vi "make step function for duty cycle.vi"(7 "delay":dbl, 8 "amplitude":dbl, 9 "period":dbl, 10 "duty cycle":dbl, 11 "sample rate":dbl) -> (3 "Waveform out":waveform(dbl))   [LabVIEW 2025]
uses:
  <vilib>/Analysis/NI_AALBase.lvlib
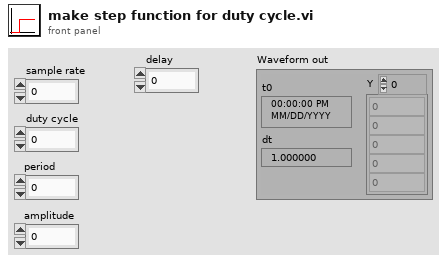
[diagram p1: front panel]
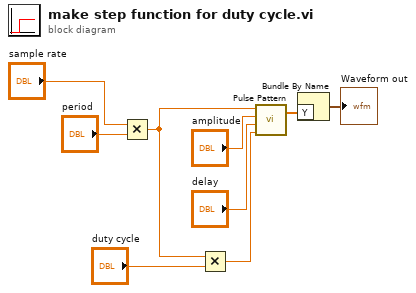
[diagram p0: block diagram]
diagram:
  n1 = Multiply(x="sample rate", y="period") -> (x*y=w1:dbl)
  n2 = Multiply(x=w1, y="duty cycle") -> (x*y=w7:dbl)
  n3 = call <vilib>:"Pulse Pattern.vi"("width"=w7, "delay"="delay", "amplitude"="amplitude", "samples"=w1) -> ("Pulse Pattern"=w9:dbl[])  [unwired: 1 out]
  n4 = Bundle By Name("Y"=w9) -> (→"Waveform out":waveform(dbl))  [unwired: 1 in]
